vi "AOL Z Cal-Sort cal array.vi"(11 "Unsorted cal":sgl[][](array[numeric])=[[0.0, 175.0, 235.0, 350.0], [0.0, 0.0, 0.1, 0.2], [1.0, 11.0, 111.0, 1111.0], [-1.0, -11.0, -111.0, -1111.0], [0.8, 88.0, 888.0, 8888.0], [-0.8, -88.0, -888.0, -8888.0], [0.6, 66.0, 667.0, 6676.0], [-0.6, -66.0, -667.0, -6676.0], [0.4, 44.0, 444.0, 4444.0], [-0.4, -44.0, -444.0, -4444.0], [0.2, 22.0, 222.0, 2222.0], [-0.2, -22.0, -222.0, -2222.0]]) -> (3 "Sorted cal":sgl[][](array[numeric]))   [LabVIEW 2020]
uses:
  <userlib>/_OpenG.lib/array/array.llb/Sort 1D Array (SGL)__ogtk.vi
  <userlib>/_OpenG.lib/array/array.llb/Reorder 2D Array2 (SGL)__ogtk.vi
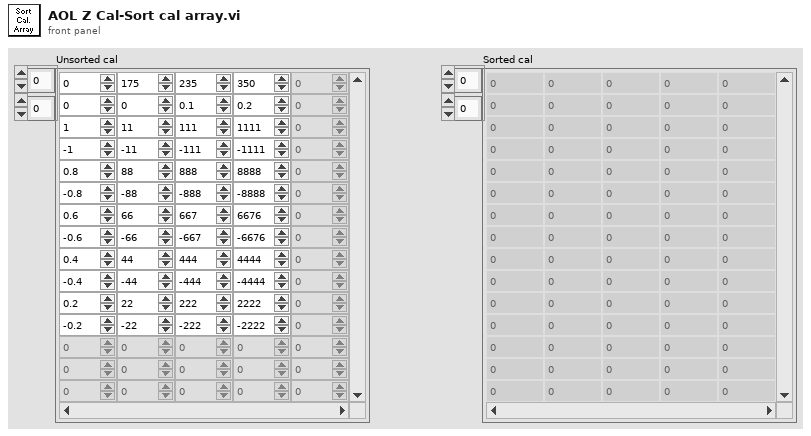
[diagram p1: front panel]
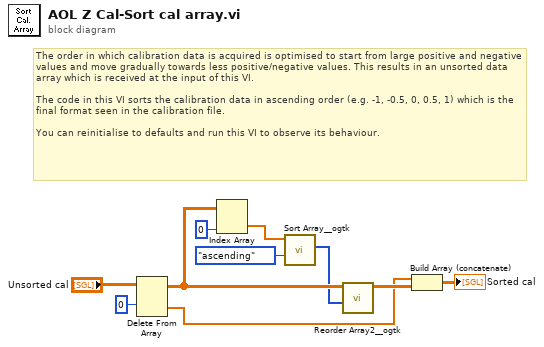
[diagram p0: block diagram]
diagram:
  # "The order in which calibration data is acquired is optimised to start from large positive and negative values and move gradually towards less positive/negative values. This results in an unsorted data array which is received at the input of this VI.\n\nThe code in this VI sorts the calibration data in ascending order (e.g. -1, -0.5, 0, 0.5, 1) which is the final format seen in the calibration file.\n\nYou can reinitialise to defaults and run this VI to observe its behaviour."
  n1 = Delete From Array(array="Unsorted cal", index (row)=0) -> (deleted portion=w1:sgl[], array with subset deleted=w5:sgl[][])  [unwired: 2 in]
  n2 = Index Array(array=w5, index (col)=0 ("disabled index (col)")) -> (element=w7:sgl[])  [unwired: 1 in]
  n3 = call-poly <userlib>:"Sort Array__ogtk.vi"("Order"=enum16{"ascending", "descending"}."ascending", "Array in"=w7) -> ("Sorted Pointers"=w4:i32[])  [unwired: 8 in, 1 out]
  n4 = call-poly <userlib>:"Reorder Array2__ogtk.vi"("indices"=w4, "array"=w5) -> ("reordered array"=w3:sgl[][])  [unwired: 9 in]
  n5 = Build Array (concatenate)(w1, w3) -> (→"Sorted cal":sgl[][])
